vi "Read Master Bounds Rect.vi"(9 "GObject in":refnum<class "GObject.lvclass">) -> (3 "GObject out":refnum<class "GObject.lvclass">, 4 "Master Bounds Rect":T1)   [LabVIEW 2014, in "GObject.lvclass"]
uses:
  GObject.lvclass
  <vilib>/Utility/miscctls.llb/LVRectTypeDef.ctl
  GObject.lvclass/GObject.ctl
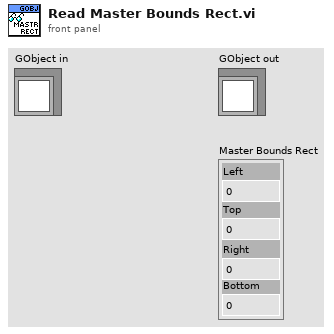
[diagram p1: front panel]
types:
  T1 = typedef "LVRectTypeDef.ctl" = cluster{"Left":i16, "Top":i16, "Right":i16, "Bottom":i16}
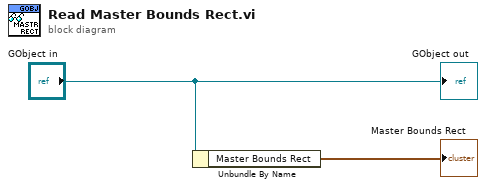
[diagram p0: block diagram]
diagram:
  n1 = Unbundle By Name("GObject in") -> ("Master Bounds Rect"=→"Master Bounds Rect":T1)
  "GObject out" <- "GObject in"
